vi "lsl resolver results.vi"(8 "error in (no error)":errorcluster, 9 "buffer_elements":u32, 10 "buffer":cluster{}, 11 "res":cluster{}) -> (0 "error out":errorcluster, 1 "function return":i32, 2 "buffer out":cluster{}, 3 "res out":cluster{})   [LabVIEW 2018, in "liblsl-LabVIEW.lvlib"]
doc: "extern LIBLSL_C_API int32_t lsl_resolver_results(lsl_continuous_resolver res, lsl_streaminfo *buffer, uint32_t buffer_elements);"
uses:
  <userlib>/liblsl-LabVIEW/liblsl-LabVIEW.lvlib
  <userlib>/liblsl-LabVIEW/liblsl64.dll
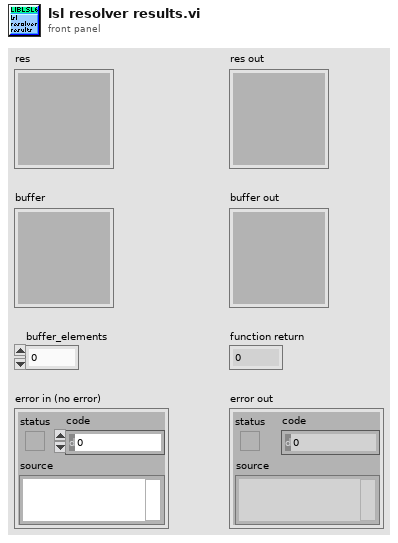
[diagram p1: front panel]
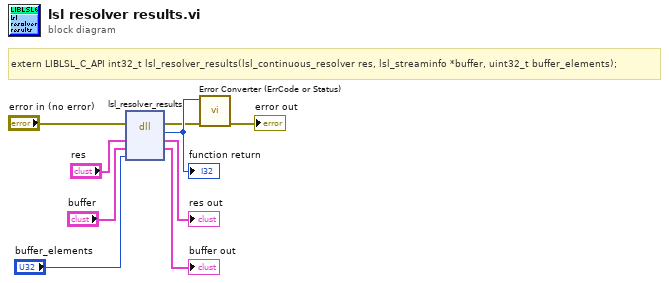
[diagram p0: block diagram]
diagram:
  # "extern LIBLSL_C_API int32_t lsl_resolver_results(lsl_continuous_resolver res, lsl_streaminfo *buffer, uint32_t buffer_elements);"
  n1 = dll-call lib="C:/Program Files/National Instruments/LabVIEW 2018/user.lib/liblsl-LabVIEW/liblsl64.*" fn="lsl_resolver_results"(error in="error in (no error)", "res"="res", "buffer"="buffer", "buffer_elements"="buffer_elements") -> (error out=w2:errorcluster, w9:i32, "res"=→"res out":cluster{}, "buffer"=→"buffer out":cluster{})  [unwired: 3 in, 1 out]
  "function return" <- w9
  n2 = call <userlib>:"Error Converter (ErrCode or Status).vi"("error in (no error)"=w2, "error code"=w9) -> ("error out"=→"error out":errorcluster)  [unwired: 9 in]
